vi "createQueues.vi"() -> (2 "Display Queue":refnum<queue>)   [LabVIEW 2017]
panel:
  in  "Image Pixels (U16)":u16[][](array[numeric])
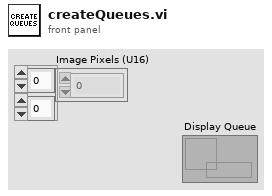
[diagram p1: front panel]
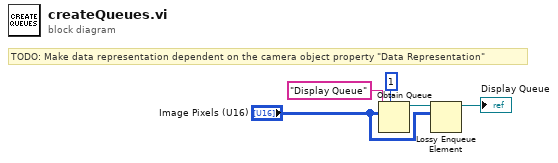
[diagram p0: block diagram]
diagram:
  # "TODO: Make data representation dependent on the camera object property \"Data Representation\""
  n1 = Obtain Queue(max queue size (-1, unlimited)=1, name (unnamed)="Display Queue", element data type="Image Pixels (U16)") -> (queue out=w3:refnum<queue>)  [unwired: 2 in, 2 out]
  n2 = Lossy Enqueue Element(queue=w3, element="Image Pixels (U16)") -> (queue out=→"Display Queue":refnum<queue>)  [unwired: 1 in, 3 out]
